vi "CIF Core UI.vi"() -> ()   [LabVIEW 2021, in "CIF Core UI.lvlib"]
uses:
  CIF Core UI.lvlib
  CIFUI/Typedef/Channel Connection.ctl
  CIFUI/Typedef/Force Channel.ctl
  CIFUI/Typedef/Core UI References.ctl
  CIFUI/CIF_UI.lvclass/CIF_UI.ctl
  CIFUI/Typedef/Direction to Include.ctl
  CIFUI/UI Element Update/Empty Tree.vi
  CIFUI/UI Element Update/Empty Table.vi
  CIFUI/CIF_UI.lvclass
panel:
  in  "Force Channel":T1
  in  "Link Channel":bool
  in  "Connection":T2
  in  "Channels":string(tree)
  in  "Connect":bool
  in  "stop":bool
  in  "address":string="192.168.1.160"
  out "Connected":bool
  in  "Clear Local":bool
  out "local error":errorcluster
  in  "Plugin Status":string[][](table)
  in  "Force":bool
  out "Current Config":string
  in  "New Config":string
  in  "Unload":bool
  in  "Refresh Button":bool
  in  "Pause":bool
  in  "Start":bool
  in  "Update Config":bool
  in  "Session Id":u64
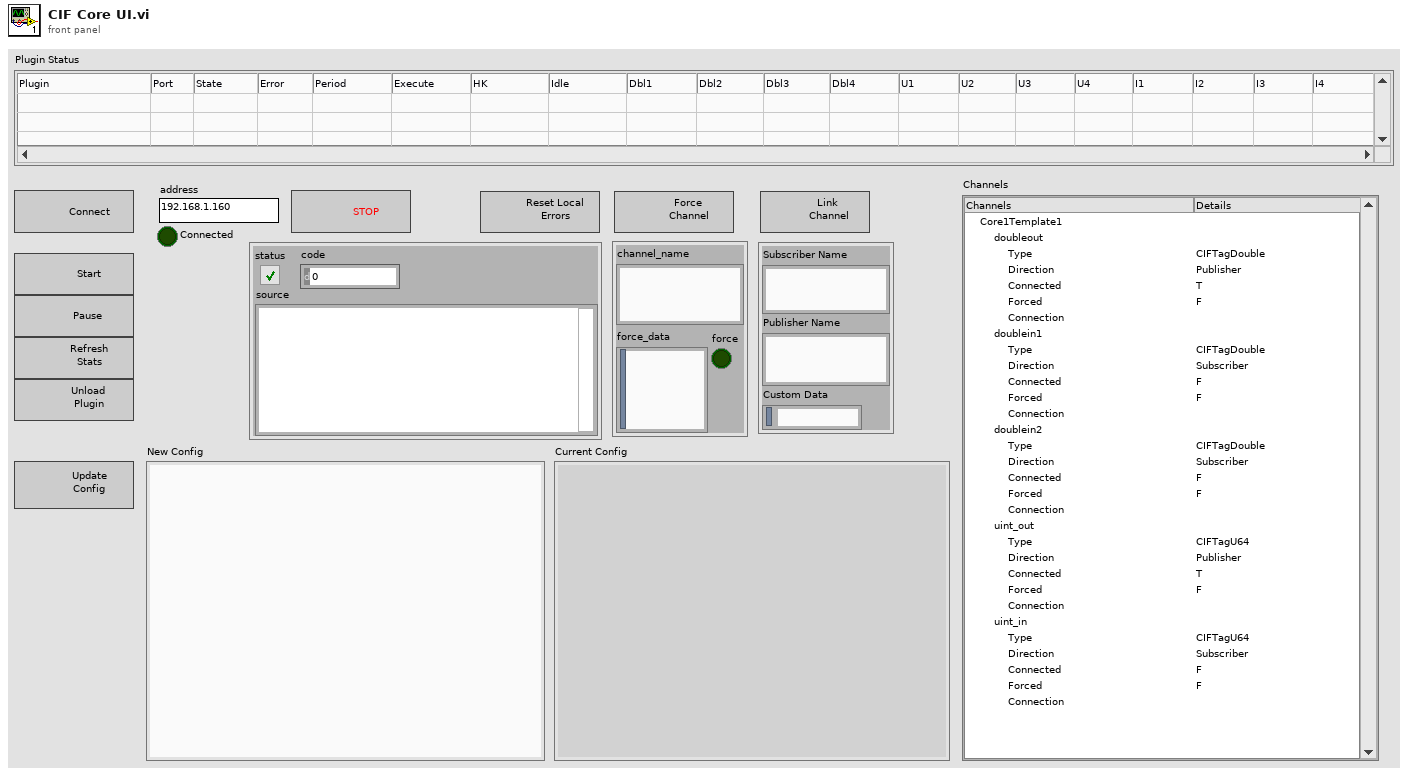
[diagram p1: front panel]
types:
  T1 = typedef "CIF_UI.lvclass/Force Channel.ctl" = cluster{"channel_name":string, "force":bool, "force_data":string}
  T2 = typedef "CIF_UI.lvclass/Channel Connection.ctl" = cluster{"Subscriber Name":string, "Publisher Name":string, "Custom Data":string}
  T3 = typedef "CIF_UI.lvclass/Core UI References.ctl" = cluster{"Discovered Plugins":refnum<vi>, "Discovered Plugins Valid":bool, "Loaded Plugins":refnum<vi>, "Loaded Plugins Valid":bool, "Publisher Channels":refnum<vi>, "Publisher Channels Valid":bool, "Subscriber Channels":refnum<vi>, "Subscriber Channels Valid":bool, "Plugin Status":refnum<vi>, "Plugin Status Valid":bool, "Channel Connection":refnum<vi>, "Channel Connection Valid":bool, "New Plugin Load":refnum<vi>, "New Plugin Load Valid":bool, "Errors":refnum<vi>, "Errors Valid":bool, "Plugin to Abort":refnum<vi>, "Plugin to Abort Valid":bool}
  T4 = typedef "InstrumentStudio Plugin SDK.lvlib/Event Registration Refnum.ctl" = refnum<event-registration>
  T5 = typedef "CIF_UI.lvclass/Direction to Include.ctl" = enum16{"All", "Subscriber", "Publisher"}
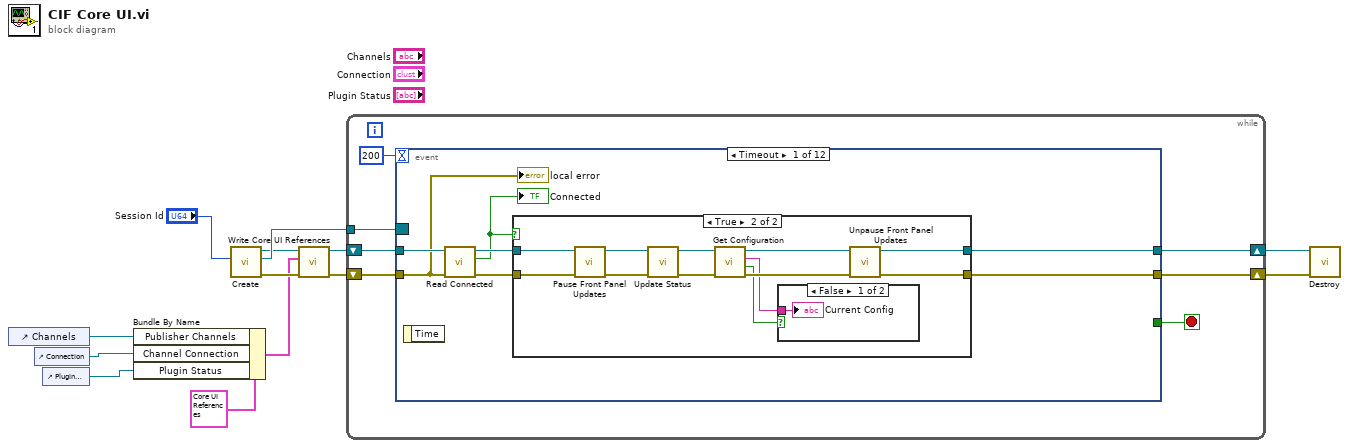
[diagram p0: block diagram]
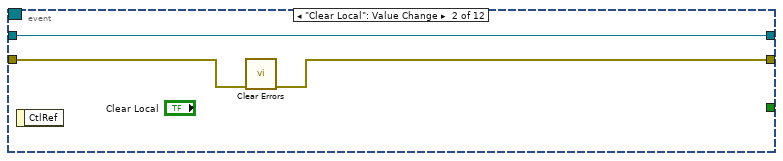
[diagram p4: hidden frame]
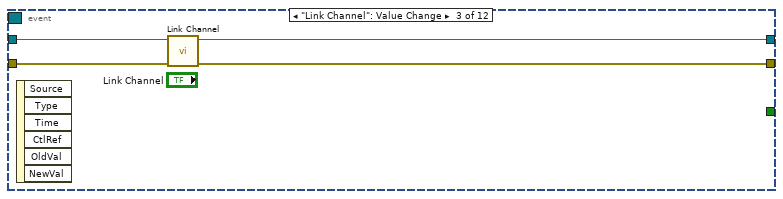
[diagram p5: hidden frame]
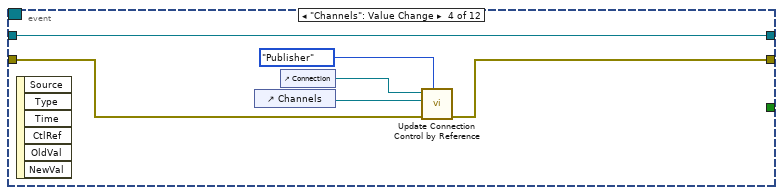
[diagram p6: hidden frame]
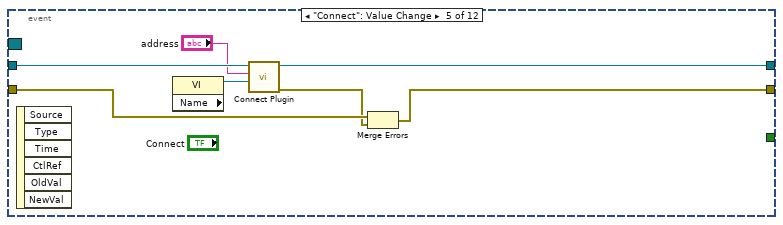
[diagram p7: hidden frame]
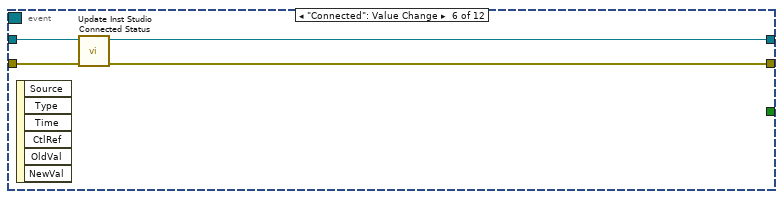
[diagram p8: hidden frame]
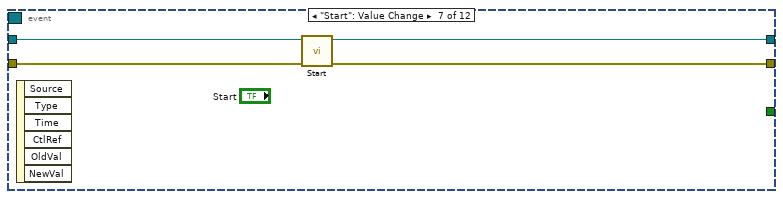
[diagram p9: hidden frame]
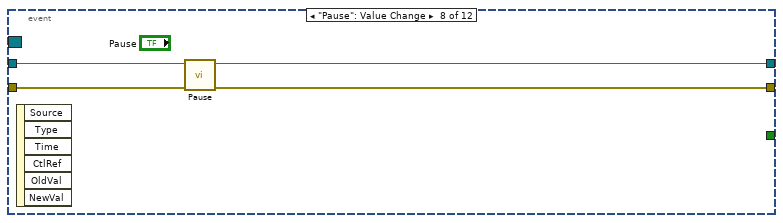
[diagram p10: hidden frame]
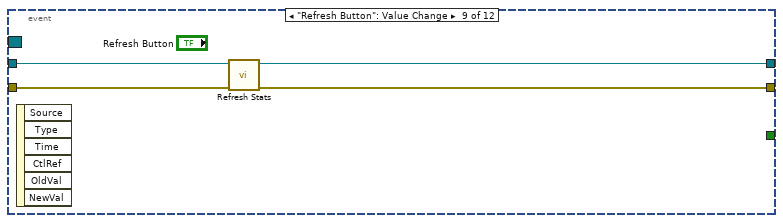
[diagram p11: hidden frame]
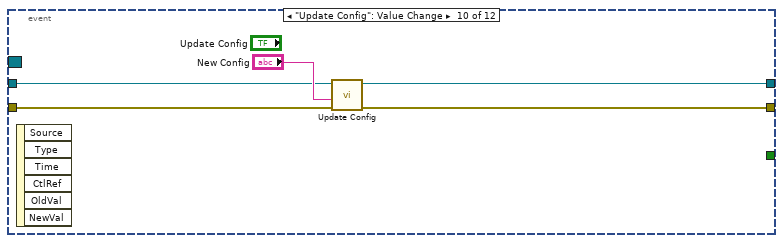
[diagram p12: hidden frame]
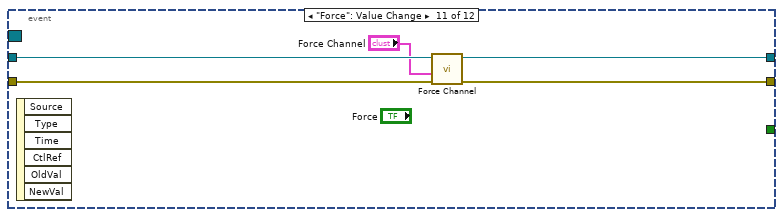
[diagram p13: hidden frame]
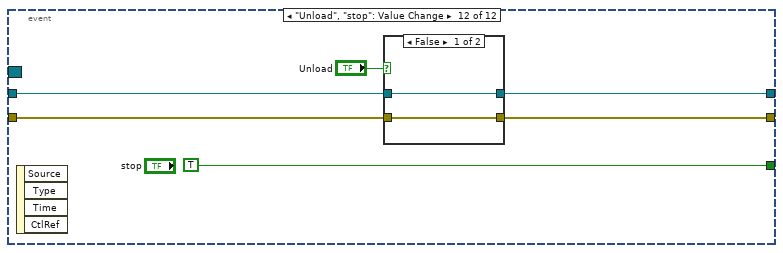
[diagram p14: hidden frame]
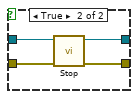
[diagram p15: hidden frame]
diagram:
  n1 = control-ref of="Channels"() -> (w11:refnum<vi>)
  n2 = control-ref of="Connection"() -> (w10:refnum<vi>)
  n3 = control-ref of="Plugin Status"() -> (w8:refnum<vi>)
  n4 = Bundle By Name(cluster=T3 {"Discovered Plugins"=refnum, "Discovered Plugins Valid"=FALSE, "Loaded Plugins"=refnum, "Loaded Plugins Valid"=FALSE, "Publisher Channels"=refnum, "Publisher Channels Valid"=FALSE, "Subscriber Channels"=refnum, "Subscriber Channels Valid"=FALSE, "Plugin Status"=refnum, "Plugin Status Valid"=FALSE, "Channel Connection"=refnum, "Channel Connection Valid"=FALSE, "New Plugin Load"=refnum, "New Plugin Load Valid"=FALSE, "Errors"=refnum, "Errors Valid"=FALSE, "Plugin to Abort"=refnum, "Plugin to Abort Valid"=FALSE} ("UI References"), "Publisher Channels"=w11, "Channel Connection"=w10, "Plugin Status"=w8) -> (w2:T3)
  n5 = call "Create.vi"("Session Id"="Session Id") -> ("error out"=w5:errorcluster, "Event Refnum"=w9:T4, "CIF_UI out"=w6:refnum<class "CIF_UI.lvclass">)  [unwired: 8 in]
  n6 = call "Write Core UI References.vi"("error in (no error)"=w5, "UI References"=w2, "CIF_UI in"=w6) -> ("error out"=w3:errorcluster, "CIF_UI out"=w4:refnum<class "CIF_UI.lvclass">)  [unwired: 7 in]
  n7 = while {
    tunnel: w9 -> [w19]
    shift-right: [w14] -> w12
    shift-left: w4 -> [w17]
    shift-right: [w15] -> w13
    shift-left: w3 -> [w16]
    stop <- w18 stop-if-true
    n8 = event shown="[0] Timeout" {
      selector: w19 -> [_ _ _ _ _ _ _ _ _ _ _ _]
      dyn-events: _ -> [_ _ _ _ _ _ _ _ _ _ _ _]
      timeout: 200 -> [_ _ _ _ _ _ _ _ _ _ _ _]
      tunnel: [_ _ _ _ _ _ _ _ _ _ _ TRUE] -> w18
      tunnel: w17 -> [w26 w43 w49 w50 w60 w66 w69 w74 w78 w82 w88 w89]
      tunnel: w16 -> [w21 w45 w48 w52 w62 w65 w70 w73 w77 w79 w87 w90]
      tunnel: [w22 w44 w47 w51 w61 w64 w67 w72 w76 w80 w85 w92] -> w15
      tunnel: [w27 w43 w46 w50 w56 w63 w68 w71 w75 w81 w86 w91] -> w14
      event Timeout {
        n9 = event-data() -> ()  [unwired: 1 in, 1 out]
        n10 = call "Read Connected.vi"("error in (no error)"=w21, "CIF_UI in"=w26) -> ("error out"=w24:errorcluster, "Connected"=w23:bool, "CIF_UI out"=w25:refnum<class "CIF_UI.lvclass">)  [unwired: 7 in]
        "Connected" <- w23
        n11 = case shown="True" w23 {
          tunnel: w24 -> [w28 w38]
          tunnel: [w28 w41] -> w22
          tunnel: w25 -> [w29 w39]
          tunnel: [w29 w40] -> w27
          frame False {
          }
          frame True {
            n12 = call "Pause Front Panel Updates.vi"("error in (no error)"=w38, "CIF_UI in"=w39) -> ("error out"=w37:errorcluster, "CIF_UI out"=w36:refnum<class "CIF_UI.lvclass">)  [unwired: 8 in]
            n13 = call "Update Status.vi"("error in (no error)"=w37, "CIF_UI in"=w36) -> ("error out"=w34:errorcluster, "CIF_UI out"=w35:refnum<class "CIF_UI.lvclass">)  [unwired: 8 in]
            n14 = call "Get Configuration.vi"("error in (no error)"=w34, "CIF_Plugin_UI in"=w35) -> ("error out"=w33:errorcluster, "Not Found"=w31:bool, "JSON Configuration"=w30:string, "CIF_Plugin_UI out"=w32:refnum<class "CIF_UI.lvclass">)  [unwired: 6 in]
            n15 = case shown="False" w31 {
              tunnel: w30 -> [w42 _]
              frame False {
                "Current Config" <- w42
              }
              frame True {
              }
            }
            n16 = call "Unpause Front Panel Updates.vi"("error in (no error)"=w33, "CIF_UI in"=w32) -> ("error out"=w41:errorcluster, "CIF_UI out"=w40:refnum<class "CIF_UI.lvclass">)  [unwired: 8 in]
          }
        }
        "local error" <- w21
      }
      event "Clear Local": Value Change {
        n17 = event-data() -> ()  [unwired: 1 in, 1 out]
        n18 = call <vilib>:"Clear Errors.vi"("error in (no error)"=w45) -> ("error out"=w44:errorcluster)  [unwired: 5 in, 1 out]
      }
      event "Link Channel": Value Change {
        n19 = event-data() -> ()  [unwired: 1 in, 6 out]
        n20 = call "Link Channel.vi"("error in (no error)"=w48, "CIF_UI in"=w49) -> ("error out"=w47:errorcluster, "CIF_UI out"=w46:refnum<class "CIF_UI.lvclass">)  [unwired: 8 in]
      }
      event "Channels": Value Change {
        n21 = event-data() -> ()  [unwired: 1 in, 6 out]
        n22 = control-ref of="Channels"() -> (w53:refnum<vi>)
        n23 = control-ref of="Connection"() -> (w54:refnum<vi>)
        n24 = call "Update Connection Control by Reference.vi"("Direction to Include"=Direction_to_Include."Publisher", "error in (no error)"=w52, "Channels"=w53, "Channel Connection"=w54) -> ("error out"=w51:errorcluster)  [unwired: 7 in]
      }
      event "Connect": Value Change {
        n25 = event-data() -> ()  [unwired: 1 in, 6 out]
        n26 = property class="VI" props=["Name"]() -> (reference out=w58:refnum<vi>)  [unwired: 2 in, 2 out]
        n27 = call "Connect Plugin.vi"("VI Reference"=w58, "Address"="address", "CIF_UI in"=w60) -> ("error out"=w57:errorcluster, "CIF_UI out"=w56:refnum<class "CIF_UI.lvclass">)  [unwired: 7 in]
        n28 = Merge Errors(w62, w57) -> (w61:errorcluster)
      }
      event "Connected": Value Change {
        n29 = event-data() -> ()  [unwired: 1 in, 6 out]
        n30 = call "Update Inst Studio Connected Status.vi"("error in (no error)"=w65, "CIF_UI in"=w66) -> ("error out"=w64:errorcluster, "CIF_UI out"=w63:refnum<class "CIF_UI.lvclass">)  [unwired: 8 in]
      }
      event "Start": Value Change {
        n31 = event-data() -> ()  [unwired: 1 in, 6 out]
        n32 = call "Start.vi"("error in (no error)"=w70, "CIF_Plugin_UI in"=w69) -> ("error out"=w67:errorcluster, "CIF_Plugin_UI out"=w68:refnum<class "CIF_UI.lvclass">)  [unwired: 7 in, 1 out]
      }
      event "Pause": Value Change {
        n33 = event-data() -> ()  [unwired: 1 in, 6 out]
        n34 = call "Pause.vi"("error in (no error)"=w73, "CIF_Plugin_UI in"=w74) -> ("error out"=w72:errorcluster, "CIF_Plugin_UI out"=w71:refnum<class "CIF_UI.lvclass">)  [unwired: 7 in, 1 out]
      }
      event "Refresh Button": Value Change {
        n35 = event-data() -> ()  [unwired: 1 in, 6 out]
        n36 = call "Refresh Stats.vi"("error in (no error)"=w77, "CIF_Plugin_UI in"=w78) -> ("error out"=w76:errorcluster, "CIF_Plugin_UI out"=w75:refnum<class "CIF_UI.lvclass">)  [unwired: 7 in, 1 out]
      }
      event "Update Config": Value Change {
        n37 = event-data() -> ()  [unwired: 1 in, 6 out]
        n38 = call "Update Config.vi"("error in (no error)"=w79, "JSON Configuration"="New Config", "CIF_Plugin_UI in"=w82) -> ("error out"=w80:errorcluster, "CIF_Plugin_UI out"=w81:refnum<class "CIF_UI.lvclass">)  [unwired: 6 in, 1 out]
      }
      event "Force": Value Change {
        n39 = event-data() -> ()  [unwired: 1 in, 6 out]
        n40 = call "Force Channel.vi"("error in (no error)"=w87, "Force Channel"="Force Channel", "CIF_Plugin_UI in"=w88) -> ("error out"=w85:errorcluster, "CIF_Plugin_UI out"=w86:refnum<class "CIF_UI.lvclass">)  [unwired: 6 in, 1 out]
      }
      event "Unload", "stop": Value Change {
        n41 = event-data() -> ()  [unwired: 1 in, 4 out]
        n42 = case shown="False" "Unload" {
          tunnel: [w96 w99] -> w91
          tunnel: [w95 w100] -> w92
          tunnel: w90 -> [w95 w98]
          tunnel: w89 -> [w96 w97]
          frame False {
          }
          frame True {
            n43 = call "Stop.vi"("error in (no error)"=w98, "CIF_Plugin_UI in"=w97) -> ("error out"=w100:errorcluster, "CIF_Plugin_UI out"=w99:refnum<class "CIF_UI.lvclass">)  [unwired: 7 in, 1 out]
          }
        }
      }
    }
  }
  n44 = call "Destroy.vi"("error in (no error)"=w13, "CIF_UI in"=w12) -> ()  [unwired: 8 in, 2 out]
